vi "Get Channel Tag Path.vi"(11 "Waveform":waveform(dbl)) -> (3 "channel path":string)   [LabVIEW 2015]
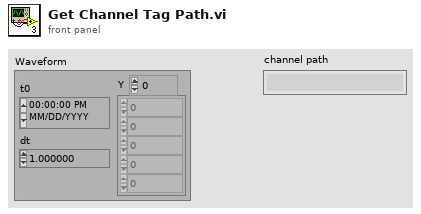
[diagram p1: front panel]
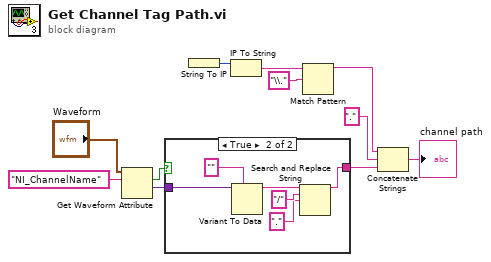
[diagram p0: block diagram]
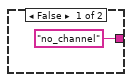
[diagram p2: hidden frame]
diagram:
  n1 = Get Waveform Attribute(6:"NI_ChannelName" ("name"), 7:"Waveform") -> (1:w10:variant, 2:w9:bool)  [unwired: 2 in, 2 out]
  n2 = case shown="True" w9 {
    tunnel: w10 -> [_ w18]
    tunnel: ["no_channel" ("result string") w15] -> w1
    frame False {
    }
    frame True {
      n3 = Variant To Data(type="" ("String"), Variant=w18) -> (data=w16:string)  [unwired: 1 in, 1 out]
      n4 = Search and Replace String(input string=w16, search string="/", replace string="." ("replace string (\"\")")) -> (result string=w15:string)  [unwired: 5 in, 3 out]
    }
  }
  n5 = String To IP() -> (0:w7:u32)  [unwired: 1 in]
  n6 = IP To String(2:w7) -> (0:w6:string)  [unwired: 1 in]
  n7 = Match Pattern(string=w6, regular expression="\\.") -> (before substring=w3:string)  [unwired: 1 in, 3 out]
  n8 = Concatenate Strings(w3, "." ("string"), w1) -> (→"channel path":string)
